vi "Find Invalid Transfer Channels.vi"(8 "error in (no error)":errorcluster, 10 "transfer ID":string, 11 "dsf refnum":T1) -> (0 "error out":errorcluster, 1 "Invalid Channels":string[](array[string]), 3 "dsf refnum out":T1, 4 "found?":bool)   [LabVIEW 2017, in "DSF Core.lvlib"]
uses:
  DSF Core.lvlib
  Controls/DSF Config Data RefNum.ctl
  Read Item Child IDs/Read Transfer Channel IDs.vi
  Read All Item IDs/Read All Channel IDs.vi
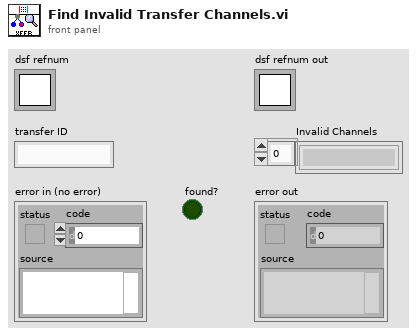
[diagram p1: front panel]
types:
  T1 = typedef "DSF Core.lvlib/DSF Config Data RefNum.ctl" = refnum<k1>
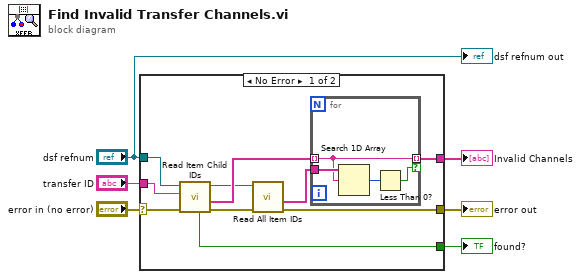
[diagram p0: block diagram]
diagram:
  n1 = case shown="No Error" "error in (no error)" {
    selector: "error in (no error)" -> [w14 w21]
    tunnel: "dsf refnum" -> [w13 _]
    tunnel: [w8 w21] -> w4
    tunnel: "transfer ID" -> [w16 _]
    tunnel: [w15 _] -> w2
    tunnel: [w10 _] -> w1
    frame No Error {
      n2 = call-poly "Read Item Child IDs.vi"("error in (no error)"=w14, "Transfer ID"=w16, "dsf refnum"=w13) -> ("error out"=w9:errorcluster, "Channel IDs"=w12:string[], "dsf refnum out"=w7:T1, "found?"=w15:bool)  [unwired: 5 in]
      n3 = call-poly "Read All Item IDs.vi"("error in (no error)"=w9, "dsf refnum"=w7) -> ("error out"=w8:errorcluster, "Channel IDs"=w11:string[])  [unwired: 7 in, 1 out]
      n4 = for {
        tunnel: w12 -> [w18] mode=indexing
        tunnel: w11 -> [w20]
        tunnel: [w18] -> w10 mode=indexing if=w17
        n5 = Search 1D Array(1D array=w20, element=w18) -> (index of element=w19:i32)  [unwired: 1 in]
        n6 = Less Than 0?(x=w19) -> (x < 0?=w17:bool)
      }
    }
    frame Error {
    }
  }
  "error out" <- w4
  "found?" <- w2
  "Invalid Channels" <- w1
  "dsf refnum out" <- "dsf refnum"
